vi "read sdf ref.vi"(8 "error in (no error)":errorcluster, 11 "abstract-tree in":refnum<class "abstract-tree.lvclass">) -> (0 "error out":errorcluster, 1 "sdf ref":refnum<k24>, 3 "abstract-tree out":refnum<class "abstract-tree.lvclass">)   [LabVIEW 2017, in "vs-tree-utility.lvlib" / "abstract-tree.lvclass"]
uses:
  abstract-tree.lvclass
  NationalInstruments.VeriStand.SystemDefinitionAPI
  abstract-tree.lvclass/abstract-tree.ctl
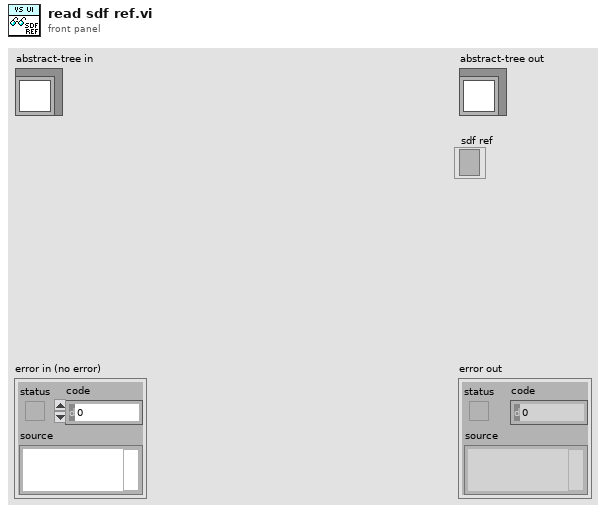
[diagram p1: front panel]
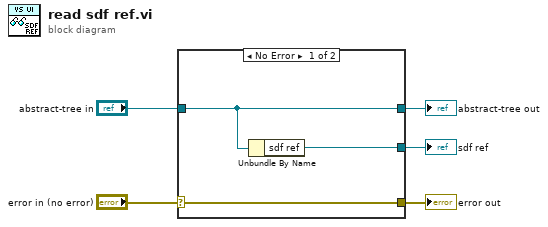
[diagram p0: block diagram]
diagram:
  n1 = case shown="No Error" "error in (no error)" {
    selector: "error in (no error)" -> [w8 w10]
    tunnel: [w8 w10] -> w4
    tunnel: [w7 w9] -> w2
    tunnel: "abstract-tree in" -> [w7 w9]
    tunnel: [w6 _] -> w1
    frame No Error {
      n2 = Unbundle By Name(w7) -> ("sdf ref"=w6:refnum<k24>)
    }
    frame Error {
    }
  }
  "error out" <- w4
  "abstract-tree out" <- w2
  "sdf ref" <- w1
